vi "Vacuum Control.vi"() -> ()   [LabVIEW 2016]
uses:
  Classes/Controller/Controller.lvclass
  Classes/Controller/I-O/I-O.lvclass
panel:
  in  "stop":bool
  in  "On/Off":bool=TRUE
  in  "Region":i32
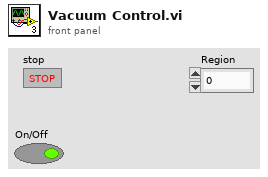
[diagram p1: front panel]
types:
  T1 = typedef "Controller.lvclass/Controllers.ctl" = cluster{"I-O.lvclass":refnum<class "I-O.lvclass">, "Motion.lvclass":refnum<class "Motion.lvclass">, "Dispenser.lvclass":refnum<class "Dispenser.lvclass">}
  T2 = typedef "I-O.lvclass/Pin Map.ctl" = cluster{"Region Valves":i32[], "Extra Valves":dbl[][][], "Tool Primary Valve":i32, "Tool Secondary Valve":i32, "Region Sensors":i32[], "Extra Sensors":dbl[][][], "Tool Primary Sensor":dbl, "Tool Secondary Sensor":dbl, "Compression Sensor":dbl, "5V":i32}
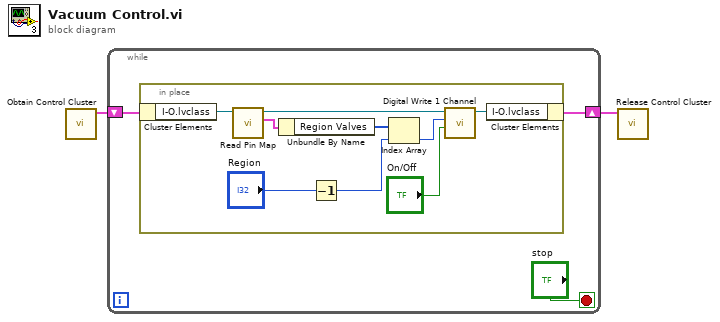
[diagram p0: block diagram]
diagram:
  n1 = call "Obtain Control Cluster.vi"() -> ("Control Out"=w2:T1)  [unwired: 11 in]
  n2 = while {
    shift-right: [w4] -> w1
    shift-left: w2 -> [w5]
    stop <- "stop" stop-if-true
    n3 = in-place {
      n4 = in-place-cluster #1(w5) -> ("I-O.lvclass"=w14:refnum<class "I-O.lvclass">)
      n5 = call-dynamic "Read Pin Map.vi"("I-O in"=w14) -> ("Pin Map 2"=w13:T2, "I-O out"=w12:refnum<class "I-O.lvclass">)  [unwired: 8 in, 1 out]
      n6 = Unbundle By Name(w13) -> ("Region Valves"=w11:i32[])
      n7 = Decrement(x="Region") -> (x-1=w9:i32)
      n8 = Index Array(array=w11, index=w9) -> (element=w8:i32)
      n9 = call-dynamic "Digital Write 1 Channel.vi"("Value"="On/Off", "Channel"=w8, "I-O.lvclass"=w12) -> ("I-O.lvclass 2"=w6:refnum<class "I-O.lvclass">)  [unwired: 7 in, 1 out]
      n10 = in-place-cluster #1("I-O.lvclass"=w6) -> (w4:T1)
    }
  }
  n11 = call "Release Control Cluster.vi"("output cluster"=w1) -> ()  [unwired: 11 in]
